vi "CMN_GetControllerStatus.vi"(11 "DBS Ref":T1) -> (1 "dhe string":string, 2 "ControllerStatus":T2={"Response"="", "power"=TRUE, "shutter"=FALSE, "artifdata"=FALSE, "idlemode"=FALSE, "reset"=FALSE, "gain"=0, "speed"=0, "resetPCI"=FALSE, "autoshutter"=FALSE, "TempSetPoint"=-110, "multipleextensions"=TRUE, "displayImage"=TRUE, "coadding"=FALSE, "images being coadded"=1, "Operation Mode"=enum."normal", "frames to write"={"subs"=FALSE, "reset"=FALSE, "exposed"=FALSE}, "fawler samples"=1, "write auto"=TRUE, "datatype"="", "frames to display"={"subs"=FALSE, "reset"=FALSE, "exposed"=FALSE}, "sur"=1, "autoclear"=TRUE})   [LabVIEW 2016]
uses:
  CMN_ContStatus.ctl
  DBSHAND/private/vis/DatabaseHand_RefNum.ctl
  DBSHAND/private/vis/DatabaseHand_Element_Get(bool).vi
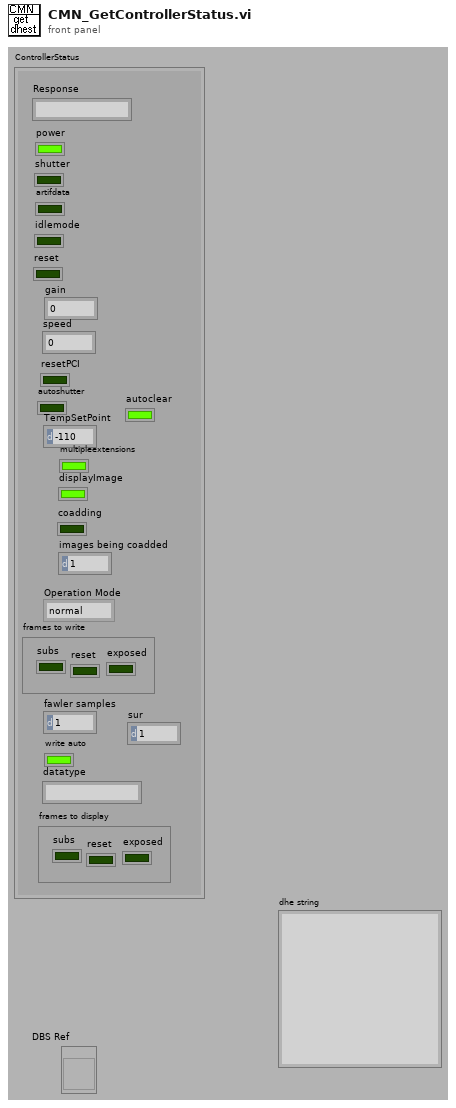
[diagram p1: front panel]
types:
  T1 = typedef "DatabaseHand_RefNum.ctl" = refnum<vi>
  T2 = typedef "CMN_ContStatus.ctl" = cluster{"Response":string, "power":bool, "shutter":bool, "artifdata":bool, "idlemode":bool, "reset":bool, "gain":u8, "speed":u8, "resetPCI":bool, "autoshutter":bool, "TempSetPoint":i32, "multipleextensions":bool, "displayImage":bool, "coadding":bool, "images being coadded":i32, "Operation Mode":enum16{"normal", "coadd", "fawler"}, "frames to write":cluster{"subs":bool, "reset":bool, "exposed":bool}, "fawler samples":i32, "write auto":bool, "datatype":string, "frames to display":cluster{"subs":bool, "reset":bool, "exposed":bool}, "sur":i32, "autoclear":bool}
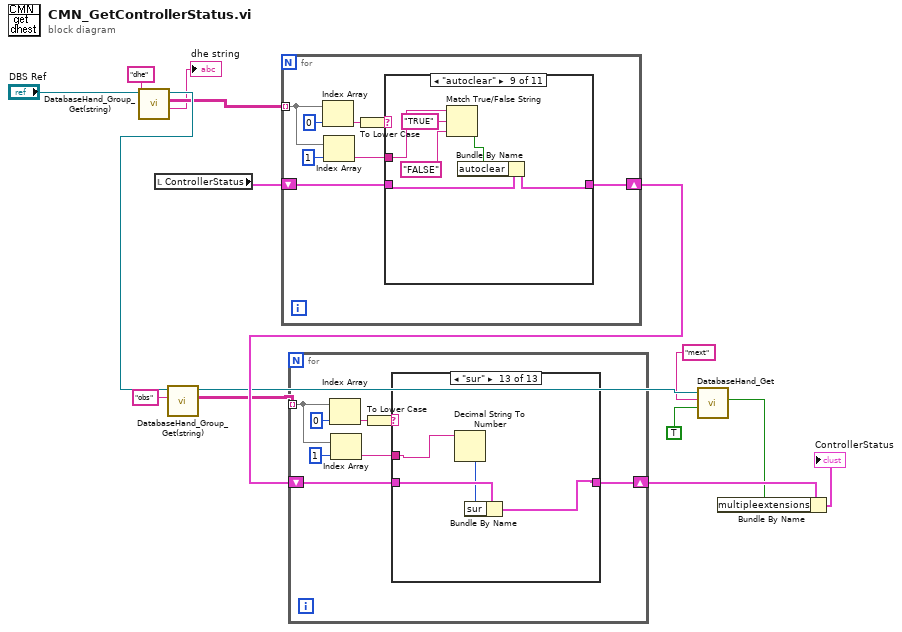
[diagram p0: block diagram]
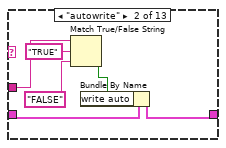
[diagram p3: hidden frame]
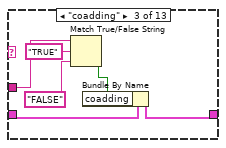
[diagram p4: hidden frame]
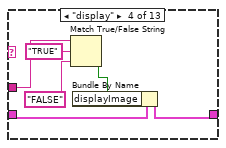
[diagram p5: hidden frame]
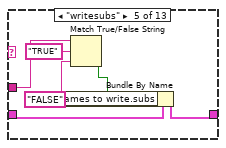
[diagram p6: hidden frame]
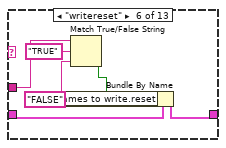
[diagram p7: hidden frame]
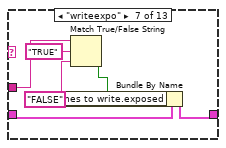
[diagram p8: hidden frame]
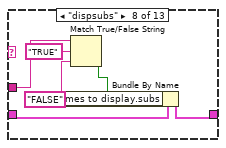
[diagram p9: hidden frame]
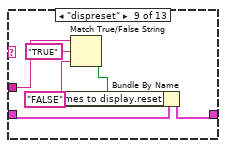
[diagram p10: hidden frame]
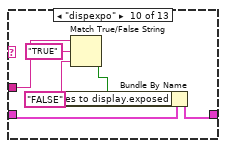
[diagram p11: hidden frame]
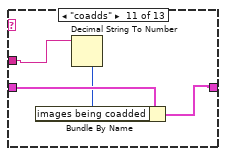
[diagram p12: hidden frame]
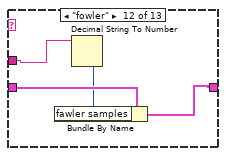
[diagram p13: hidden frame]
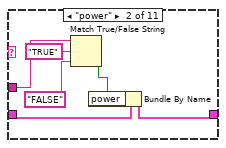
[diagram p15: hidden frame]
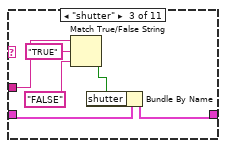
[diagram p16: hidden frame]
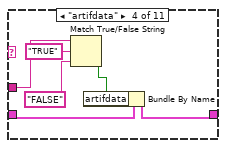
[diagram p17: hidden frame]
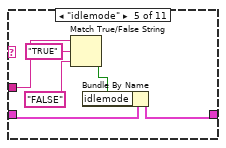
[diagram p18: hidden frame]
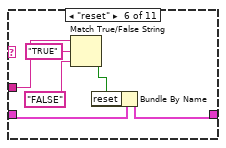
[diagram p19: hidden frame]
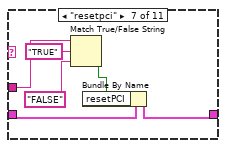
[diagram p20: hidden frame]
diagram:
  n1 = call "DatabaseHand_Group_Get(string).vi"("group"="dhe", "Database RefNum in"="DBS Ref") -> ("group string"=→"dhe string":string, "group array"=w3:string[][], "Database RefNum out"=w12:T1)  [unwired: 1 in, 6 out]
  n2 = local read "ControllerStatus"() -> (w14:T2)
  n3 = call "DatabaseHand_Group_Get(string).vi"("group"="obs", "Database RefNum in"=w12) -> ("group array"=w4:string[][], "Database RefNum out"=w10:T1)  [unwired: 1 in, 7 out]
  n4 = for {
    tunnel: w3 -> [w18] mode=indexing
    shift-right: [w20] -> w13
    shift-left: w14 -> [w21]
    n5 = Index Array(array=w18, index=0) -> (element=w22:string)
    n6 = Index Array(array=w18, index=1) -> (element=w17:string)
    n7 = To Lower Case(string=w22) -> (all lower case string=w16:string)
    n8 = case shown="\"autoclear\"" w16 {
      tunnel: w21 -> [w24 w30 w36 w42 w48 w54 w60 w66 w72 w76 w80]
      tunnel: [w24 w29 w35 w41 w47 w53 w59 w65 w71 w73 w79] -> w20
      tunnel: w17 -> [_ w28 w34 w40 w46 w52 w58 w64 w70 w75 w78]
      frame Default {
      }
      frame "power" {
        n9 = Match True/False String(2:"FALSE" ("false string"), 3:"TRUE" ("true string"), 4:w28) -> (0:w27:bool)  [unwired: 1 out]
        n10 = Bundle By Name(cluster=w30, "power"=w27) -> (w29:T2)
      }
      frame "shutter" {
        n11 = Match True/False String(2:"FALSE" ("false string"), 3:"TRUE" ("true string"), 4:w34) -> (0:w33:bool)  [unwired: 1 out]
        n12 = Bundle By Name(cluster=w36, "shutter"=w33) -> (w35:T2)
      }
      frame "artifdata" {
        n13 = Match True/False String(2:"FALSE" ("false string"), 3:"TRUE" ("true string"), 4:w40) -> (0:w39:bool)  [unwired: 1 out]
        n14 = Bundle By Name(cluster=w42, "artifdata"=w39) -> (w41:T2)
      }
      frame "idlemode" {
        n15 = Match True/False String(2:"FALSE" ("false string"), 3:"TRUE" ("true string"), 4:w46) -> (0:w45:bool)  [unwired: 1 out]
        n16 = Bundle By Name(cluster=w48, "idlemode"=w45) -> (w47:T2)
      }
      frame "reset" {
        n17 = Match True/False String(2:"FALSE" ("false string"), 3:"TRUE" ("true string"), 4:w52) -> (0:w51:bool)  [unwired: 1 out]
        n18 = Bundle By Name(cluster=w54, "reset"=w51) -> (w53:T2)
      }
      frame "resetpci" {
        n19 = Match True/False String(2:"FALSE" ("false string"), 3:"TRUE" ("true string"), 4:w58) -> (0:w57:bool)  [unwired: 1 out]
        n20 = Bundle By Name(cluster=w60, "resetPCI"=w57) -> (w59:T2)
      }
      frame "autoshutter" {
        n21 = Match True/False String(2:"FALSE" ("false string"), 3:"TRUE" ("true string"), 4:w64) -> (0:w63:bool)  [unwired: 1 out]
        n22 = Bundle By Name(cluster=w66, "autoshutter"=w63) -> (w65:T2)
      }
      frame "autoclear" {
        n23 = Match True/False String(2:"FALSE" ("false string"), 3:"TRUE" ("true string"), 4:w70) -> (0:w69:bool)  [unwired: 1 out]
        n24 = Bundle By Name(cluster=w72, "autoclear"=w69) -> (w71:T2)
      }
      frame "gain" {
        n25 = Decimal String To Number(string=w75, default (0L)=u8 0) -> (number=w77:u8)  [unwired: 2 out]
        n26 = Bundle By Name(cluster=w76, "gain"=w77) -> (w73:T2)
      }
      frame "speed" {
        n27 = Decimal String To Number(string=w78) -> (number=w81:i32)  [unwired: 3 out]
        n28 = Bundle By Name(cluster=w80, "speed"=w81) -> (w79:T2)
      }
    }
  }
  n29 = for {
    tunnel: w4 -> [w84] mode=indexing
    shift-right: [w86] -> w8
    shift-left: w13 -> [w87]
    n30 = Index Array(array=w84, index=0) -> (element=w88:string)
    n31 = Index Array(array=w84, index=1) -> (element=w83:string)
    n32 = To Lower Case(string=w88) -> (all lower case string=w82:string)
    n33 = case shown="\"sur\"" w82 {
      tunnel: w87 -> [w90 w96 w102 w108 w114 w120 w126 w132 w138 w144 w148 w152 w156]
      tunnel: [w90 w95 w101 w107 w113 w119 w125 w131 w137 w143 w147 w151 w155] -> w86
      tunnel: w83 -> [_ w94 w100 w106 w112 w118 w124 w130 w136 w142 w146 w150 w154]
      frame Default {
      }
      frame "autowrite" {
        n34 = Match True/False String(2:"FALSE" ("false string"), 3:"TRUE" ("true string"), 4:w94) -> (0:w93:bool)  [unwired: 1 out]
        n35 = Bundle By Name(cluster=w96, "write auto"=w93) -> (w95:T2)
      }
      frame "coadding" {
        n36 = Match True/False String(2:"FALSE" ("false string"), 3:"TRUE" ("true string"), 4:w100) -> (0:w99:bool)  [unwired: 1 out]
        n37 = Bundle By Name(cluster=w102, "coadding"=w99) -> (w101:T2)
      }
      frame "display" {
        n38 = Match True/False String(2:"FALSE" ("false string"), 3:"TRUE" ("true string"), 4:w106) -> (0:w105:bool)  [unwired: 1 out]
        n39 = Bundle By Name(cluster=w108, "displayImage"=w105) -> (w107:T2)
      }
      frame "writesubs" {
        n40 = Match True/False String(2:"FALSE" ("false string"), 3:"TRUE" ("true string"), 4:w112) -> (0:w111:bool)  [unwired: 1 out]
        n41 = Bundle By Name(cluster=w114, "frames to write.subs"=w111) -> (w113:T2)
      }
      frame "writereset" {
        n42 = Match True/False String(2:"FALSE" ("false string"), 3:"TRUE" ("true string"), 4:w118) -> (0:w117:bool)  [unwired: 1 out]
        n43 = Bundle By Name(cluster=w120, "frames to write.reset"=w117) -> (w119:T2)
      }
      frame "writeexpo" {
        n44 = Match True/False String(2:"FALSE" ("false string"), 3:"TRUE" ("true string"), 4:w124) -> (0:w123:bool)  [unwired: 1 out]
        n45 = Bundle By Name(cluster=w126, "frames to write.exposed"=w123) -> (w125:T2)
      }
      frame "dispsubs" {
        n46 = Match True/False String(2:"FALSE" ("false string"), 3:"TRUE" ("true string"), 4:w130) -> (0:w129:bool)  [unwired: 1 out]
        n47 = Bundle By Name(cluster=w132, "frames to display.subs"=w129) -> (w131:T2)
      }
      frame "dispreset" {
        n48 = Match True/False String(2:"FALSE" ("false string"), 3:"TRUE" ("true string"), 4:w136) -> (0:w135:bool)  [unwired: 1 out]
        n49 = Bundle By Name(cluster=w138, "frames to display.reset"=w135) -> (w137:T2)
      }
      frame "dispexpo" {
        n50 = Match True/False String(2:"FALSE" ("false string"), 3:"TRUE" ("true string"), 4:w142) -> (0:w141:bool)  [unwired: 1 out]
        n51 = Bundle By Name(cluster=w144, "frames to display.exposed"=w141) -> (w143:T2)
      }
      frame "coadds" {
        n52 = Decimal String To Number(string=w146) -> (number=w145:i32)  [unwired: 3 out]
        n53 = Bundle By Name(cluster=w148, "images being coadded"=w145) -> (w147:T2)
      }
      frame "fowler" {
        n54 = Decimal String To Number(string=w150) -> (number=w149:i32)  [unwired: 3 out]
        n55 = Bundle By Name(cluster=w152, "fawler samples"=w149) -> (w151:T2)
      }
      frame "sur" {
        n56 = Decimal String To Number(string=w154) -> (number=w153:i32)  [unwired: 3 out]
        n57 = Bundle By Name(cluster=w156, "sur"=w153) -> (w155:T2)
      }
    }
  }
  n58 = call-poly "DatabaseHand_Get.vi"("default value"=TRUE, "name"="mext", "Database RefNum in"=w10) -> ("value"=w5:bool)  [unwired: 2 in, 6 out]
  n59 = Bundle By Name(cluster=w8, "multipleextensions"=w5) -> (→"ControllerStatus":T2)
